vi "DAC Init.vi"(7 "WaveDataNum":u16, 9 "pWaveData":u16[](array[numeric])=array[4097 elements], 10 "CycleUs":u16, 11 "DevHandle":i32) -> (1 "pWaveData out":u16[](array[numeric]), 3 "function return":i32)   [LabVIEW 2010, in "usb2dac.lvlib"]
doc: "int WINAPI DAC_Init(int DevHandle,unsigned short CycleUs,unsigned short *pWaveData,unsigned short WaveDataNum);"
uses:
  usb2dac.lvlib
  USB2XXX/trunk/USB2XXX/USB2XXX/vs2010/Release/USB2XXX.dll
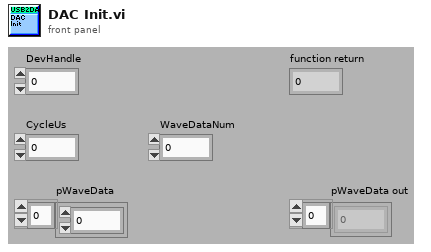
[diagram p1: front panel]
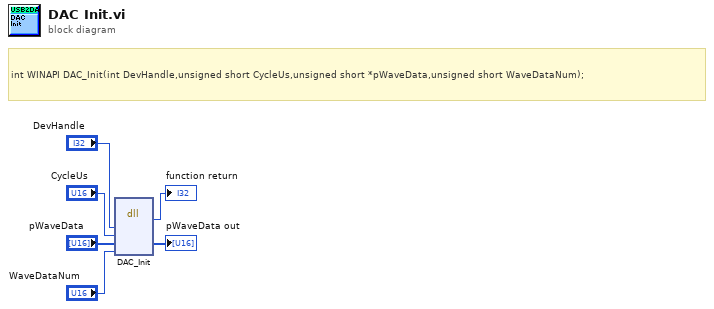
[diagram p0: block diagram]
diagram:
  # "int WINAPI DAC_Init(int DevHandle,unsigned short CycleUs,unsigned short *pWaveData,unsigned short WaveDataNum);"
  n1 = dll-call lib="E:/Projects/USB2XXX/trunk/USB2XXX/USB2XXX/vs2010/Release/USB2XXX.*" fn="DAC_Init"("DevHandle"="DevHandle", "CycleUs"="CycleUs", "pWaveData"="pWaveData", "WaveDataNum"="WaveDataNum") -> (→"function return":i32, "pWaveData"=→"pWaveData out":u16[])  [unwired: 6 in, 2 out]
